vi "TPNPT_Filter.vi"(0 "Values":dbl[](array[numeric]) format="%.2f", 1 "last value":dbl format="%.2f", 2 "Number of samples":i32, 4 "index":i32, 5 "filter":string) -> (7 "output":dbl format="%.2f", 8 "Values out":dbl[](array[numeric]) format="%.2f")   [LabVIEW 2016]
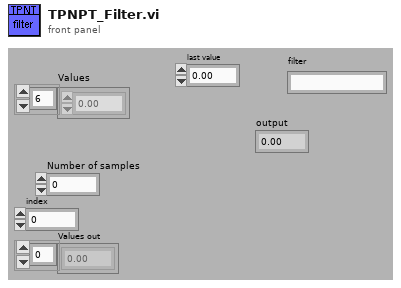
[diagram p1: front panel]
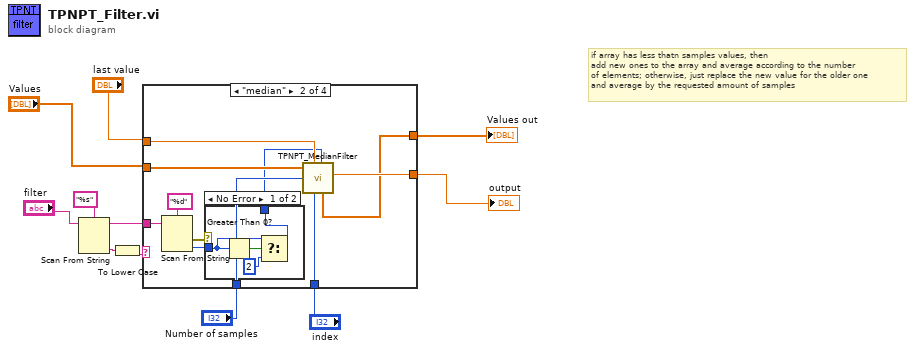
[diagram p0: block diagram]
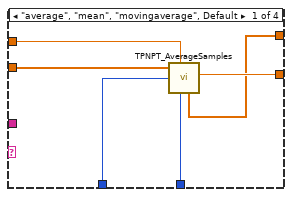
[diagram p2: hidden frame]
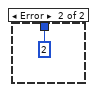
[diagram p3: hidden frame]
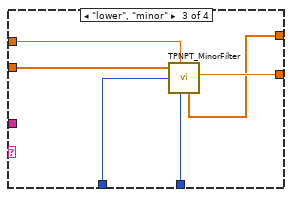
[diagram p4: hidden frame]
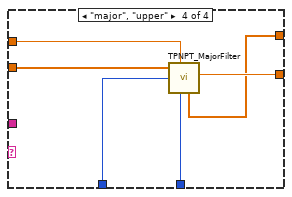
[diagram p5: hidden frame]
diagram:
  # "if array has less thatn samples values, then\nadd new ones to the array and average according to the number\nof elements; otherwise, just replace the new value for the older one\nand average by the requested amount of samples"
  n1 = Scan From String(format string="%s", input string="filter") -> (remaining string=w1:string, output 1=w3:string)  [unwired: 2 in, 3 out]
  n2 = To Lower Case(string=w3) -> (all lower case string=w2:string)
  n3 = case shown="\"median\"" w2 {
    tunnel: "Values" -> [w17 w28 w39 w45]
    tunnel: "last value" -> [w16 w27 w38 w44]
    tunnel: "Number of samples" -> [w15 w26 w37 w43]
    tunnel: "index" -> [w14 w25 w36 w42]
    tunnel: [w13 w24 w35 w41] -> w7
    tunnel: [w12 w23 w34 w40] -> w6
    tunnel: w1 -> [_ w22 _ _]
    frame "average", "mean", "movingaverage", Default {
      n4 = call "TPNPT_AverageSamples.vi"("Values"=w17, "last value"=w16, "Number of samples"=w15, "index"=w14) -> ("average"=w13:dbl, "Values out"=w12:dbl[])  [unwired: 5 out]
    }
    frame "median" {
      n5 = Scan From String(format string="%d", input string=w22) -> (error out=w20:errorcluster, output 1=w18:i32)  [unwired: 2 in, 3 out]
      n6 = case shown="No Error" w20 {
        tunnel: [w30 2] -> w19
        tunnel: w18 -> [w31 _]
        frame No Error {
          n7 = Greater Than 0?(x=w31) -> (x > 0?=w32:bool)
          n8 = Select(t=w31, s=w32, f=2) -> (s? t:f=w30:i32)
        }
        frame Error {
        }
      }
      n9 = call "TPNPT_MedianFilter.vi"("Values"=w28, "last value"=w27, "Number of samples"=w26, "index"=w25, "rank"=w19) -> ("average"=w24:dbl, "Values out"=w23:dbl[])  [unwired: 4 out]
    }
    frame "lower", "minor" {
      n10 = call "TPNPT_MinorFilter.vi"("Values"=w39, "last value"=w38, "Number of samples"=w37, "index"=w36) -> ("average"=w35:dbl, "Values out"=w34:dbl[])  [unwired: 5 out]
    }
    frame "major", "upper" {
      n11 = call "TPNPT_MajorFilter.vi"("Values"=w45, "last value"=w44, "Number of samples"=w43, "index"=w42) -> ("average"=w41:dbl, "Values out"=w40:dbl[])  [unwired: 5 out]
    }
  }
  "output" <- w7
  "Values out" <- w6
